vi "ClusterFuctions.vi"() -> ()   [LabVIEW 2018]
panel:
  out "boolean":bool
  out "num":i32
  out "string":string
  out "output cluster":T1
  in  "Boolean":bool
  in  "String":string
  in  "Numeric":i32
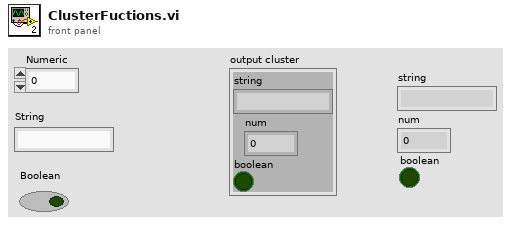
[diagram p1: front panel]
types:
  T1 = cluster{"string":string, "num":i32, "boolean":bool}
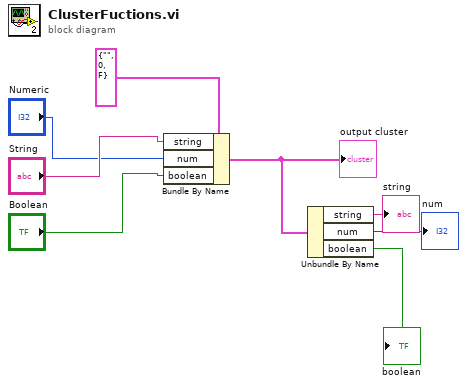
[diagram p0: block diagram]
diagram:
  n1 = Bundle By Name(cluster=T1 {"string"="", "num"=0, "boolean"=FALSE} ("input cluster"), "string"="String", "num"="Numeric", "boolean"="Boolean") -> (w4:T1)
  "output cluster" <- w4
  n2 = Unbundle By Name(w4) -> ("string"=→"string":string, "num"=→"num":i32, "boolean"=→"boolean":bool)
